vi "Check Position and Moving flag.vi"(8 "error in (no error)":errorcluster, 9 "Device Name":string, 10 "Axis Active":bool, 11 "VISA Refnum in":refnum<visa-resource-name>) -> (0 "error out":errorcluster, 2 "MovingFlag":bool, 3 "Numeric":i32)   [LabVIEW 2015]
uses:
  MCode_LV_86/Get Parameter.ctl
  MCode_LV_86/MDrive Mode.ctl
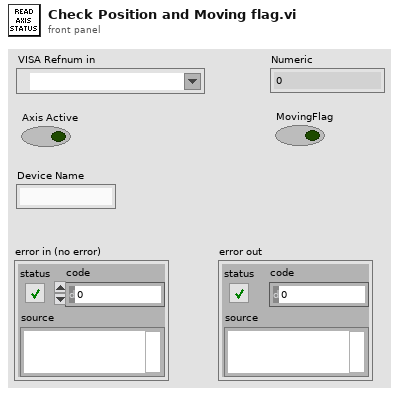
[diagram p1: front panel]
types:
  T1 = typedef "Get Parameter.ctl" = enum16{"Acceleration (A)", "Baud Rate (BD)", "Busy Flag (BY)", "Counter 1 (C1)", "Counter 2 (C2)", "Check Sum Enable (CK)", "Clock Mode (CM)", "Clock Mode Ratio (CR)", "Clock Mode Out Step Width (CW)", "Deceleration (D)", "Digital Filtering, Input 1 (D1)", "Digital Filtering, Input 2 (D2)", "Digital Filtering, Input 3 (D3)", "Digital Filtering, Input 4 (D4)", "Digital Filtering, Input 5 (D5)", "Digital Filtering, Input 9 (D9)", "Digital Filtering, Input 10 (D10)", "Digital Filtering, Input 11 (D11)", "Digital Filtering, Input 12 (D12)", "Deadband (DB)", "Enable/Disable Drive (DE)", "Device Name (DN)", "End Program Execution (E)", "Encoder Function Enable (EE)", "Encoder Lines (EL)", "Error Flag (EF)", "Error Variable (ER)", "Echo Mode (EM)", "Escape (ES)", "Execute Program at Address (EX)", "Hold Current (HC)", "Hold Current Delay Time (HI)", "Input 1 (I1)", "Input 2 (I2)", "Input 3 (I3)", "Input 4 (I4)", "Input 5 Analog (I5)", "Input 6 Encoder Index (I6)", "Input 9 (I9)", "Input 10 (I10)", "Input 11 (I11)", "Input 12 (I12)", "Input Low Byte (1-4) (IL)", "Input High Byte (9-12) (IH)", "Inputs Total (1-4,9-12) (IN)", "Internal Temperature (IT)", "Jog Enable (JE)", "Limit Stop Mode (LM)", "MicroStepping Select (MS)", "Motor Settling Delay Time (MT)", "Moving Flag (MV)", "Output 1 (O1)", "Output 2 (O2)", "Output 3 (O3)", "Output 4 (O4)", "Output 9 (O9)", "Output 10 (O10)", "Output 11 (O11)", "Output 12 (O12)", "Output High Byte (9-12) (OH)", "Output Low Byte (1-4) (OL)", "Output Total (1-4 and 9-12) (OT)", "Position (P)", "Position Captured at Trip (PC)", "Position Maintenance (PM)", "Part Number (PN)", "Party Mode (PY)", "Register 1 (R1)", "Register 2 (R2)", "Register 3 (R3)", "Register 4 (R4)", "Run Current (RC)", "Serial Number (SN)", "Stall Flag (ST)", "Stall Factor (SF)", "Stall Mode Set (SM)", "User Variables (UV)", "Velocity (V)", "Velocity Changing Flag (VC)", "Velocity Initial (VI)", "Version, Firmware (VR)", "Velocity Maximum (VM)", "Read Input1", "Read Input2"}
  T2 = typedef "MDrive Mode.ctl" = enum16{"Normal Mode", "Party Mode"}
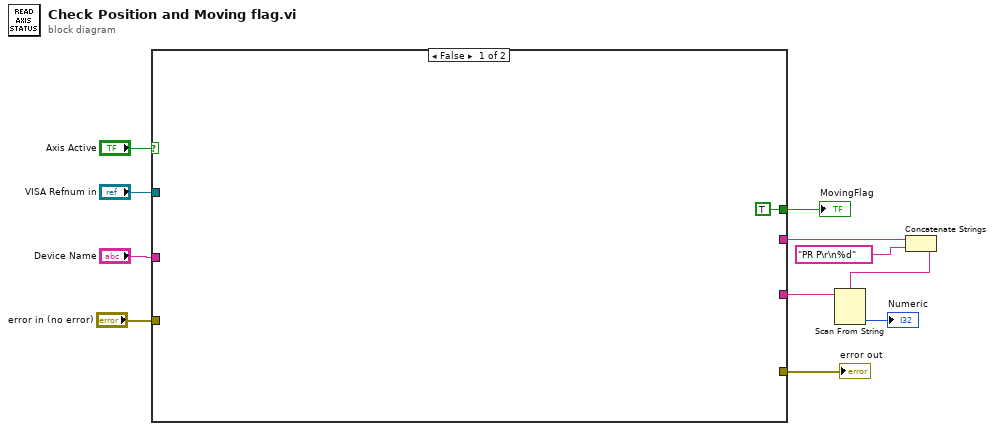
[diagram p0: block diagram]
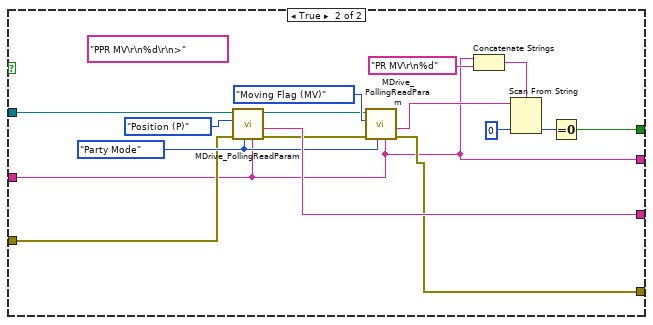
[diagram p2: hidden frame]
diagram:
  n1 = case shown="False" "Axis Active" {
    tunnel: "VISA Refnum in" -> [_ w24]
    tunnel: [_ w23] -> w9
    tunnel: [TRUE w26] -> w7
    tunnel: "Device Name" -> [_ w13]
    tunnel: [_ w15] -> w5
    tunnel: "error in (no error)" -> [_ w14]
    tunnel: [_ w13] -> w3
    frame False {
    }
    frame True {
      w17 = MDrive_Mode."Party Mode" ("Mdrive Mode")
      (unwired) "PPR MV\r\n%d\r\n>" ("format string")
      n2 = call "MDrive_PollingReadParam.vi"("Device Name"=w13, "Mdrive Mode"=w17, "error in (no error)"=w14, "Get Parameter"=Get_Parameter."Position (P)", "VISA Refnum in"=w24) -> ("error out"=w16:errorcluster, "String"=w23:string, "VISA Refnum out"=w21:refnum<visa-resource-name>)  [unwired: 3 in, 1 out]
      n3 = call "MDrive_PollingReadParam.vi"("Device Name"=w13, "Mdrive Mode"=w17, "error in (no error)"=w16, "Get Parameter"=Get_Parameter."Moving Flag (MV)", "VISA Refnum in"=w21) -> ("error out"=w15:errorcluster, "String"=w27:string)  [unwired: 3 in, 2 out]
      n4 = Concatenate Strings(w13, "PR MV\r\n%d" ("format string")) -> (w19:string)
      n5 = Scan From String(format string=w19, input string=w27, default 1=0 ("output 1")) -> (output 1=w28:i32)  [unwired: 2 in, 3 out]
      n6 = Equal To 0?(x=w28) -> (x = 0?=w26:bool)
    }
  }
  "MovingFlag" <- w7
  "error out" <- w5
  n7 = Concatenate Strings(w3, "PR P\r\n%d" ("format string")) -> (w1:string)
  n8 = Scan From String(format string=w1, input string=w9) -> (output 1=→"Numeric":i32)  [unwired: 3 in, 3 out]
